vi "数据记录.vi"(11 "写入字段":string) -> (3 "连接的字符串":string)   [LabVIEW 2016, in "数据传输系统-06.lvlib"]
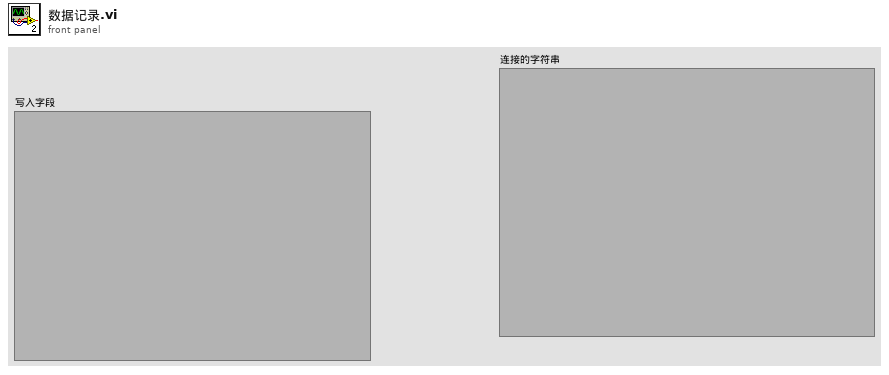
[diagram p1: front panel]
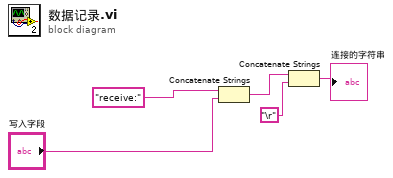
[diagram p0: block diagram]
diagram:
  n1 = Concatenate Strings("receive:" ("字符串"), "写入字段") -> (w3:string)
  n2 = Concatenate Strings(w3, "\r") -> (→"连接的字符串":string)
